vi "ReadVoltage.vi"(8 "error in (no error)":errorcluster, 11 "reference in":refnum<class "VdKeySightMM-A1.lvclass">) -> (0 "error out":errorcluster, 2 "Voltage":dbl, 3 "reference out":refnum<class "VdKeySightMM-A1.lvclass">)   [LabVIEW 2020, in "MulitMeters.lvlib" / "VdKeySightMM-A1.lvclass"]
uses:
  VdKeySightMM-A1.lvclass
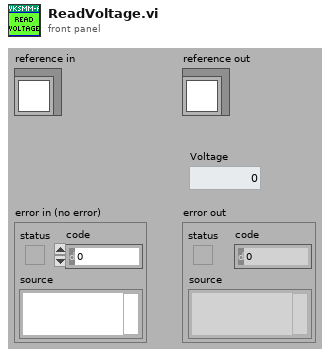
[diagram p1: front panel]
types:
  T1 = typedef "MulitMeters.lvlib/VdKeySightMM-A1.lvclass/ObjectAttributes.ctl" = cluster{"VdTcpIP":refnum<class "VdTcpIP.lvclass">}
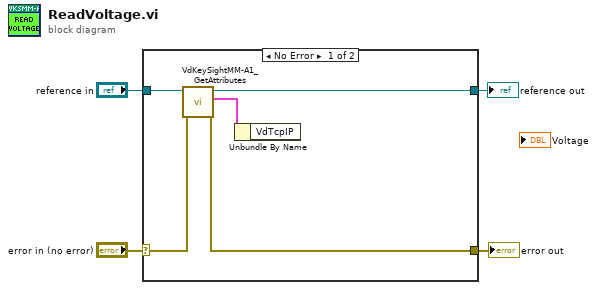
[diagram p0: block diagram]
diagram:
  n1 = case shown="No Error" "error in (no error)" {
    selector: "error in (no error)" -> [w9 w11]
    tunnel: [w7 w11] -> w3
    tunnel: [w5 w10] -> w1
    tunnel: "reference in" -> [w6 w10]
    frame No Error {
      n2 = call "VdKeySightMM-A1_GetAttributes.vi"("error in (no error)"=w9, "reference in"=w6) -> ("error out"=w7:errorcluster, "Data"=w8:T1, "reference out"=w5:refnum<class "VdKeySightMM-A1.lvclass">)  [unwired: 6 in, 1 out]
      n3 = Unbundle By Name(w8) -> ()  [unwired: 1 out]
    }
    frame Error {
    }
  }
  "error out" <- w3
  "reference out" <- w1
